vi "non-HT Subcarrier to Frequency Offset Index.vi"(9 "subcarrier index":u8, 10 "primary channel selector":fxp<+,2,2>) -> (1 "frequency offset index":fxp<+/-,9,9>)   [LabVIEW 2020]
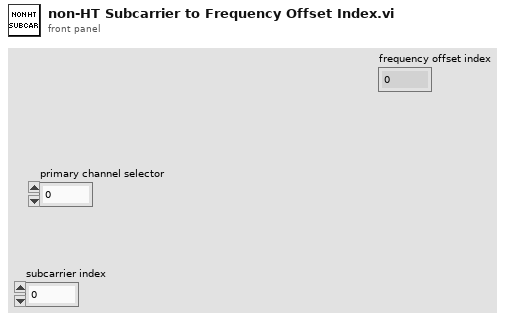
[diagram p1: front panel]
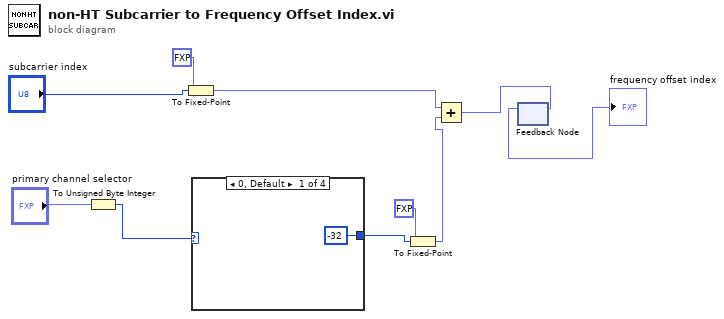
[diagram p0: block diagram]
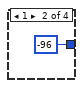
[diagram p2: hidden frame]
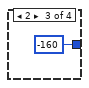
[diagram p3: hidden frame]
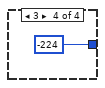
[diagram p4: hidden frame]
diagram:
  n1 = To Unsigned Byte Integer(number="primary channel selector") -> (unsigned 8bit integer=w9:u8)
  n2 = To Fixed-Point(fixed-point type=fxp<+,8,8> 0.0, number="subcarrier index") -> (fixed-point=w3:fxp<+,8,8>)
  n3 = case shown="0, Default" w9 {
    tunnel: [i16 -32 i16 -96 i16 -160 i16 -224] -> w5
    frame 0, Default {
    }
    frame 1 {
    }
    frame 2 {
    }
    frame 3 {
    }
  }
  n4 = To Fixed-Point(fixed-point type=fxp<+/-,16,16> 0.0, number=w5) -> (fixed-point=w4:fxp<+/-,16,16>)
  n5 = Add(x=w3, y=w4) -> (x+y=w2:fxp<+/-,9,9>)
  n6 = feedback-in #1(w2) -> ()
  n7 = feedback #1() -> (→"frequency offset index":fxp<+/-,9,9>)  [unwired: 1 in]
